vi "TecellaTCP.vi"(8 "error in (no error)":errorcluster, 10 "data in":string="GET /help/map.htm HTTP/1.1\nHost: www.ni.com\n\n", 11 "TecellaClient in":refnum<class "TecellaClient.lvclass">) -> (0 "error out":errorcluster, 2 "Data Returned":string, 3 "TecellaClient out":refnum<class "TecellaClient.lvclass">)   [LabVIEW 2009, in "TecellaClient.lvclass"]
uses:
  TecellaClient.lvclass
  TecellaClient.lvclass/TecellaClient.ctl
panel:
  out "Port":dbl
  out "Address":string
  in  "mode (standard)":T1(ring)=enum."CRLF"
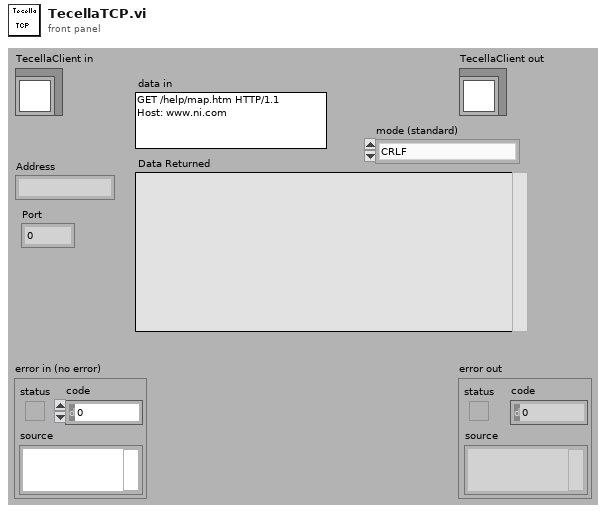
[diagram p1: front panel]
types:
  T1 = enum16{"Standard", "Buffered", "CRLF", "Immediate"}
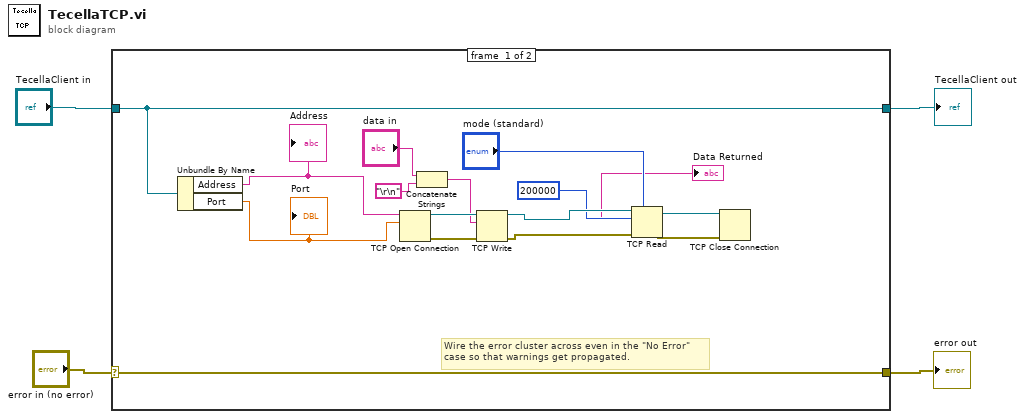
[diagram p0: block diagram]
diagram:
  n1 = case shown="No Error" "error in (no error)" {
    selector: "error in (no error)" -> [w20 w22]
    tunnel: [w20 w22] -> w3
    tunnel: [w5 w21] -> w1
    tunnel: "TecellaClient in" -> [w5 w21]
    frame #0 {
      # "Wire the error cluster across even in the \"No Error\"\ncase so that warnings get propagated."
      n2 = Unbundle By Name(w5) -> ("Address"=w7:string, "Port"=w6:dbl)
      "Address" <- w7
      "Port" <- w6
      n3 = TCP Open Connection(address=w7, remote port or service name=w6) -> (connection ID=w19:refnum<k5>, error out=w18:errorcluster)  [unwired: 3 in]
      n4 = Concatenate Strings("data in", "\r\n") -> (w13:string)
      n5 = TCP Write(connection ID=w19, data in=w13, error in (no error)=w18) -> (connection ID out=w11:refnum<k5>, error out=w10:errorcluster)  [unwired: 1 in, 1 out]
      n6 = TCP Read(connection ID=w11, bytes to read=200000, error in (no error)=w10, 7:"mode (standard)") -> (connection ID out=w17:refnum<k5>, data out=→"Data Returned":string, error out=w16:errorcluster)  [unwired: 1 in]
      n7 = TCP Close Connection(connection ID=w17, error in (no error)=w16) -> ()  [unwired: 1 in, 2 out]
    }
    frame #1 {
    }
  }
  "error out" <- w3
  "TecellaClient out" <- w1
